vi "Draw Infrared Frame.vi"(8 "Error In":errorcluster, 10 "U16 Array":u8[](array[numeric]), 11 "Image":T1) -> (0 "Error Out":errorcluster, 3 "Image Out":T1)   [LabVIEW 2014, in "LVH-KinectOne.lvlib"]
doc: "Converts the Infrared data to a Greyscale U16 IMAQ Image."
uses:
  LVH-KinectOne.lvlib
  <vilib>/vision/Image Controls.llb/IMAQ Image.ctl
  Private/Frame Description FGV [Infrared].vi
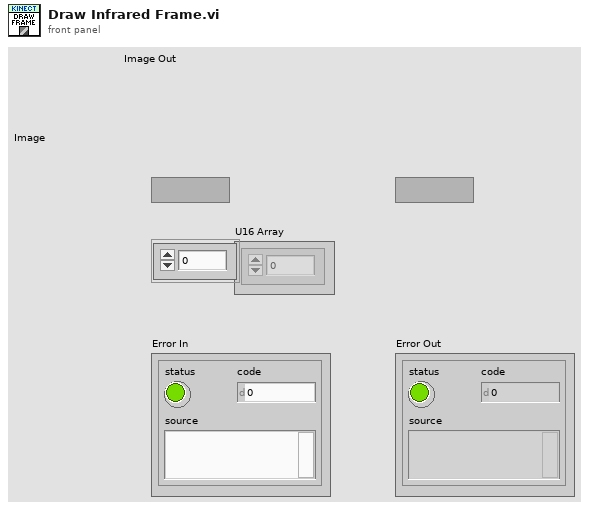
[diagram p1: front panel]
types:
  T1 = typedef "IMAQ Image.ctl" = refnum<image>
  T2 = typedef "LVH-KinectOne.lvlib/FrameDescription.ctl" = cluster{"BytesPerPixel":u32, "DiagonalFieldOfView":sgl, "Height":i32, "HorizontalFieldOfView":sgl, "LengthInPixels":u32, "VerticalFieldOfView":sgl, "Width":i32}
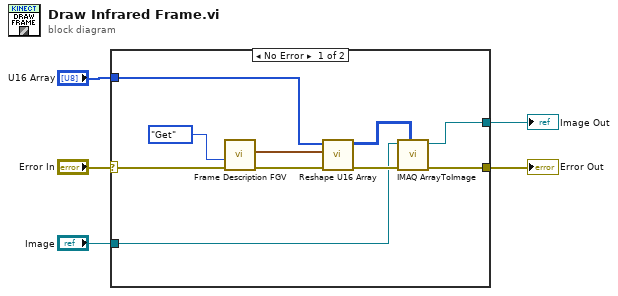
[diagram p0: block diagram]
diagram:
  n1 = case shown="No Error" "Error In" {
    selector: "Error In" -> [w6 w17]
    tunnel: "U16 Array" -> [w15 _]
    tunnel: [w10 w17] -> w1
    tunnel: "Image" -> [w8 w16]
    tunnel: [w7 w16] -> w4
    frame No Error {
      n2 = call-poly "Frame Description FGV.vi"("error in (no error)"=w6, "Command"=enum16{"Get", "Set"}."Get") -> ("error out"=w14:errorcluster, "FrameDescription"=w12:T2)  [unwired: 8 in]
      n3 = call "Reshape U16 Array.vi"("error in (no error)"=w14, "FrameDescription"=w12, "U16 Array"=w15) -> ("error out"=w11:errorcluster, "2D Array"=w9:u16[][])  [unwired: 7 in]
      n4 = call "IMAQ ArrayToImage"("Image Pixels (U16)"=w9, "error in (no error)"=w11, "Image"=w8) -> ("error out"=w10:errorcluster, "Image Out"=w7:T1)  [unwired: 7 in]
    }
    frame Error {
      # "Pass out upstream error"
    }
  }
  "Image Out" <- w4
  "Error Out" <- w1
